vi "DataXML loadXmlProcess.vi"(5 "target name":string, 7 "level":u8, 8 "error in (no error)":errorcluster, 11 "xml_data_path":path) -> (0 "error IO":errorcluster, 1 "type":string[](array[string]), 2 "value":string[](array[string]), 3 "name":string[](array[string]))   [LabVIEW 2018, in "DataXML.lvclass"]
uses:
  DataXML.lvclass
  <vilib>/xml/Load XML File.vi
  <vilib>/Utility/error.llb/Error Cluster From Error Code.vi
  <vilib>/ErrorRing/Error Ring.xnode
  <vilib>/xml/NI_XML.lvlib
  <resource>/objmgr/DOMUserDefRef.rc
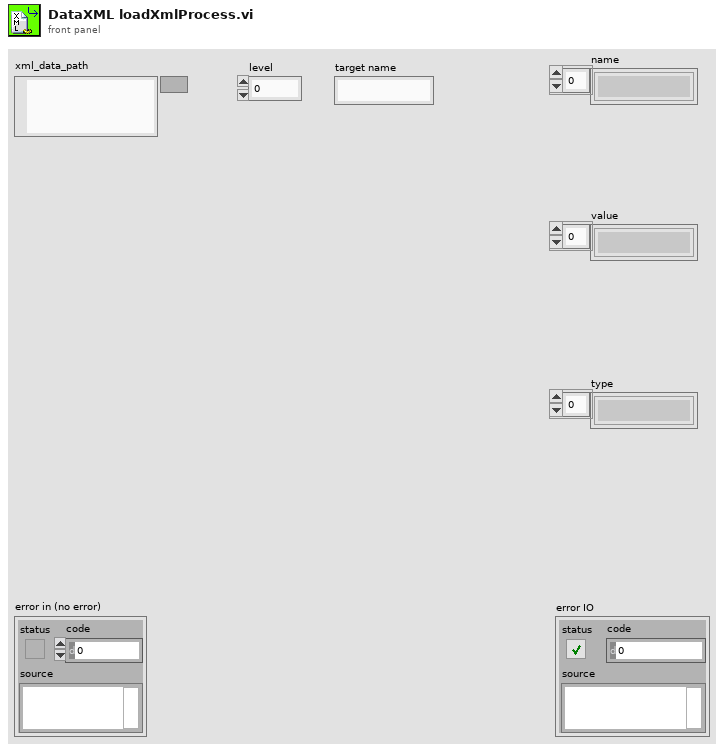
[diagram p1: front panel]
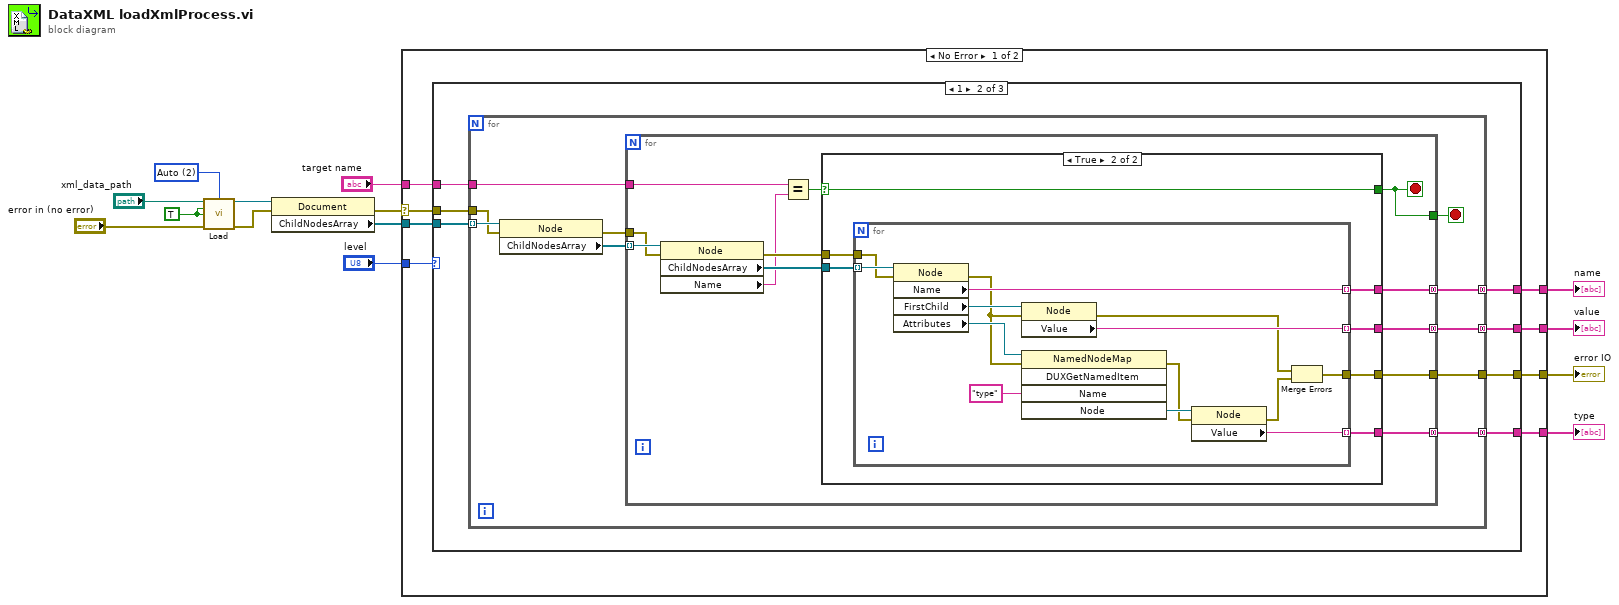
[diagram p0: block diagram]
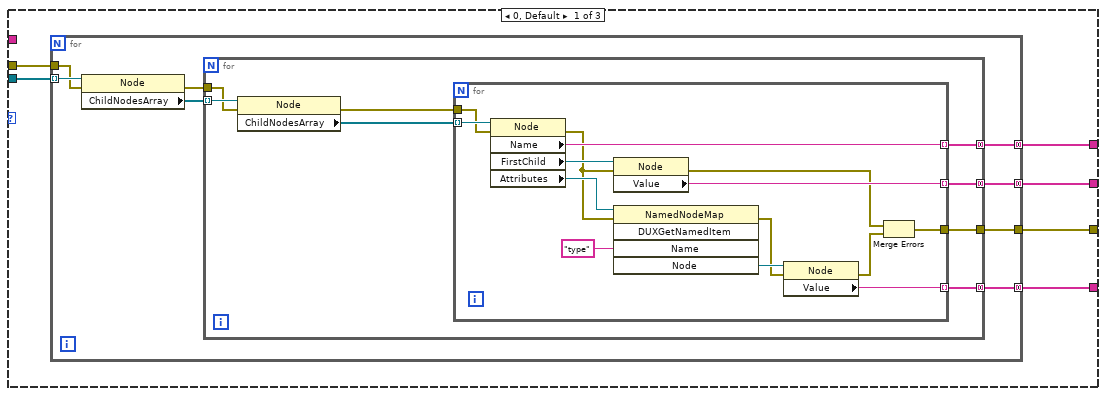
[diagram p2: hidden frame]
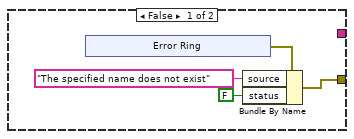
[diagram p3: hidden frame]
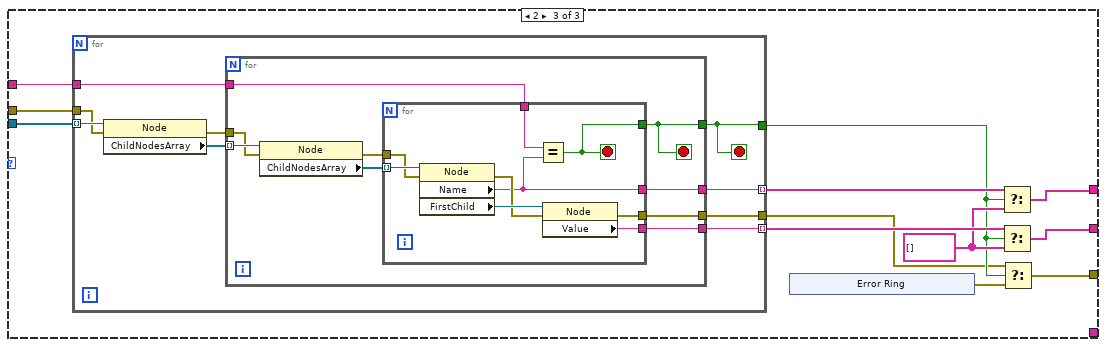
[diagram p4: hidden frame]
diagram:
  w13 = 2 items=["Never", "Always", "Auto"] ("validate on load (Auto)")
  w14 = TRUE ("process namespaces (False)")
  n1 = call-poly <vilib>:"Load.vi"("path to XML document"="xml_data_path", "validate on load (Auto)"=w13, "process namespaces (False)"=w14, "process schema (False)"=w14, "error in (no error)"="error in (no error)") -> ("DOM document out"=w12:refnum<k20>, "error out"=w10:errorcluster)  [unwired: 8 in, 1 out]
  n2 = property class="Document"(reference=w12, error in=w10) -> (error out=w1:errorcluster, "ChildNodesArray"=w6:refnum<k20>[])  [unwired: 1 out]
  n3 = case shown="No Error" w1 {
    selector: w1 -> [w15 w160]
    tunnel: "level" -> [w22 _]
    tunnel: "target name" -> [w21 _]
    tunnel: w6 -> [w20 _]
    tunnel: [w19 _] -> w5
    tunnel: [w18 _] -> w4
    tunnel: [w17 w160] -> w3
    tunnel: [w16 _] -> w2
    frame No Error {
      n4 = case shown="1" w22 {
        tunnel: w21 -> [_ w59 w126]
        tunnel: w15 -> [w28 w65 w128]
        tunnel: w20 -> [w27 w64 w127]
        tunnel: [w26 w63 w122] -> w19
        tunnel: [w25 w62 w121] -> w18
        tunnel: [w24 w61 _] -> w16
        tunnel: [w23 w60 w118] -> w17
        frame 0, Default {
          n5 = for {
            tunnel: w27 -> [w36] mode=indexing
            tunnel: [w34] -> w26 mode=concatenating
            tunnel: [w33] -> w24 mode=concatenating
            tunnel: [w32] -> w25 mode=concatenating
            tunnel: w28 -> [w31]
            tunnel: [w29] -> w23
            n6 = property class="Node"(reference=w36, error in=w31) -> (error out=w30:errorcluster, "ChildNodesArray"=w35:refnum<k20>[])  [unwired: 1 out]
            n7 = for {
              tunnel: w35 -> [w44] mode=indexing
              tunnel: [w42] -> w34 mode=concatenating
              tunnel: [w41] -> w33 mode=concatenating
              tunnel: [w40] -> w32 mode=concatenating
              tunnel: w30 -> [w39]
              tunnel: [w37] -> w29
              n8 = property class="Node"(reference=w44, error in=w39) -> (error out=w38:errorcluster, "ChildNodesArray"=w43:refnum<k20>[])  [unwired: 1 out]
              n9 = for {
                tunnel: w43 -> [w58] mode=indexing
                tunnel: [w57] -> w42 mode=indexing
                tunnel: [w54] -> w41 mode=indexing
                tunnel: [w51] -> w40 mode=indexing
                tunnel: w38 -> [w50]
                tunnel: [w45] -> w37
                n10 = property class="Node"(reference=w58, error in=w50) -> (error out=w49:errorcluster, "Name"=w57:string, "FirstChild"=w52:refnum<k20>, "Attributes"=w53:refnum<k20>)  [unwired: 1 out]
                n11 = property class="Node"(reference=w52, error in=w49) -> (error out=w46:errorcluster, "Value"=w51:string)  [unwired: 1 out]
                n12 = invoke class="NamedNodeMap" method="DUXGetNamedItem"(reference=w53, error in=w49, "Name"="type") -> (error out=w48:errorcluster, "Node"=w55:refnum<k20>)  [unwired: 2 in, 3 out]
                n13 = property class="Node"(reference=w55, error in=w48) -> (error out=w47:errorcluster, "Value"=w54:string)  [unwired: 1 out]
                n14 = Merge Errors(w46, w47) -> (w45:errorcluster)
              }
            }
          }
        }
        frame 1 {
          n15 = for {
            tunnel: w64 -> [w75] mode=indexing
            tunnel: [w73] -> w63 mode=concatenating
            tunnel: [w72] -> w61 mode=concatenating
            tunnel: [w71] -> w62 mode=concatenating
            tunnel: w65 -> [w70]
            tunnel: [w68] -> w60
            tunnel: w59 -> [w67]
            stop <- w66 stop-if-true
            n16 = property class="Node"(reference=w75, error in=w70) -> (error out=w69:errorcluster, "ChildNodesArray"=w74:refnum<k20>[])  [unwired: 1 out]
            n17 = for {
              tunnel: w74 -> [w87] mode=indexing
              tunnel: [w85] -> w73 mode=concatenating
              tunnel: [w84] -> w72 mode=concatenating
              tunnel: [w83] -> w71 mode=concatenating
              tunnel: w69 -> [w82]
              tunnel: [w80] -> w68
              tunnel: w67 -> [w79]
              tunnel: [w76] -> w66
              stop <- w76 stop-if-true
              n18 = property class="Node"(reference=w87, error in=w82) -> (error out=w81:errorcluster, "ChildNodesArray"=w86:refnum<k20>[], "Name"=w78:string)  [unwired: 1 out]
              n19 = Equal?(x=w79, y=w78) -> (x = y?=w77:bool)
              n20 = case shown="True" w77 {
                selector: w77 -> [_ w96]
                tunnel: w86 -> [_ w102]
                tunnel: [_ w101] -> w85
                tunnel: [_ w100] -> w84
                tunnel: [_ w99] -> w83
                tunnel: w81 -> [_ w98]
                tunnel: [w89 w97] -> w80
                tunnel: [_ w96] -> w76
                frame False {
                  n21 = xnode "Error Ring"() -> ("error out"=w91:errorcluster)
                  n22 = Bundle By Name(cluster=w91, "source"="The specified name does not exist", "status"=FALSE) -> (w89:errorcluster)
                }
                frame True {
                  n23 = for {
                    tunnel: w102 -> [w116] mode=indexing
                    tunnel: [w115] -> w101 mode=indexing
                    tunnel: [w112] -> w100 mode=indexing
                    tunnel: [w109] -> w99 mode=indexing
                    tunnel: w98 -> [w108]
                    tunnel: [w103] -> w97
                    n24 = property class="Node"(reference=w116, error in=w108) -> (error out=w107:errorcluster, "Name"=w115:string, "FirstChild"=w110:refnum<k20>, "Attributes"=w111:refnum<k20>)  [unwired: 1 out]
                    n25 = property class="Node"(reference=w110, error in=w107) -> (error out=w104:errorcluster, "Value"=w109:string)  [unwired: 1 out]
                    n26 = invoke class="NamedNodeMap" method="DUXGetNamedItem"(reference=w111, error in=w107, "Name"="type") -> (error out=w106:errorcluster, "Node"=w113:refnum<k20>)  [unwired: 2 in, 3 out]
                    n27 = property class="Node"(reference=w113, error in=w106) -> (error out=w105:errorcluster, "Value"=w112:string)  [unwired: 1 out]
                    n28 = Merge Errors(w104, w105) -> (w103:errorcluster)
                  }
                }
              }
            }
          }
        }
        frame 2 {
          w123 = string[] [] ("f")
          n29 = for {
            tunnel: w127 -> [w141] mode=indexing
            tunnel: w128 -> [w139]
            tunnel: [w137] -> w124 mode=indexing
            tunnel: [w136] -> w119
            tunnel: w126 -> [w135]
            tunnel: [w134] -> w125 mode=indexing
            tunnel: [w133] -> w120
            stop <- w133 stop-if-true
            n30 = property class="Node"(reference=w141, error in=w139) -> (error out=w138:errorcluster, "ChildNodesArray"=w140:refnum<k20>[])  [unwired: 1 out]
            n31 = for {
              tunnel: w140 -> [w150] mode=indexing
              tunnel: w138 -> [w148]
              tunnel: [w142] -> w137
              tunnel: [w146] -> w136
              tunnel: w135 -> [w145]
              tunnel: [w144] -> w133
              tunnel: [w143] -> w134
              stop <- w144 stop-if-true
              n32 = property class="Node"(reference=w150, error in=w148) -> (error out=w147:errorcluster, "ChildNodesArray"=w149:refnum<k20>[])  [unwired: 1 out]
              n33 = for {
                tunnel: w149 -> [w159] mode=indexing
                tunnel: [w157] -> w142
                tunnel: w147 -> [w156]
                tunnel: [w154] -> w146
                tunnel: w145 -> [w153]
                tunnel: [w152] -> w144
                tunnel: [w151] -> w143
                stop <- w152 stop-if-true
                n34 = property class="Node"(reference=w159, error in=w156) -> (error out=w155:errorcluster, "Name"=w151:string, "FirstChild"=w158:refnum<k20>)  [unwired: 1 out]
                n35 = Equal?(x=w153, y=w151) -> (x = y?=w152:bool)
                n36 = property class="Node"(reference=w158, error in=w155) -> (error out=w154:errorcluster, "Value"=w157:string)  [unwired: 1 out]
              }
            }
          }
          n37 = xnode "Error Ring"() -> ("error out"=w117:errorcluster)
          n38 = Select(t=w125, s=w120, f=w123) -> (s? t:f=w122:string[])
          n39 = Select(t=w124, s=w120, f=w123) -> (s? t:f=w121:string[])
          n40 = Select(t=w119, s=w120, f=w117) -> (s? t:f=w118:errorcluster)
        }
      }
    }
    frame Error {
    }
  }
  "name" <- w5
  "value" <- w4
  "error IO" <- w3
  "type" <- w2
